vi "Lambda Flow Auto (Read).vi"(6 "ISOBUS address":T5=-1 caption="ISOBUS address (-1)", 8 "error in":errorcluster, 11 "Mercury Reference In":T2) -> (0 "error out":errorcluster, 2 "Lambda Auto":string, 3 "Mercury Reference Out":T2, 4 "Valid?":T1)   [LabVIEW 2016, in "Mercury iXX.lvlib" / "Lambda.lvlib"]
doc: "Check if the flow of the control loop is in automatic mode."
uses:
  Lambda.lvlib
  Controls/Mercury Reference.ctl
  Controls/Comms Transport Layer.ctl
  Private/Controls/Query Dynamic Reference.ctl
  Controls/ISOBus Address.ctl
  Controls/Is Valid LED.ctl
  Private/Controls/Command Verbs.ctl
  Mercury iXX.lvlib
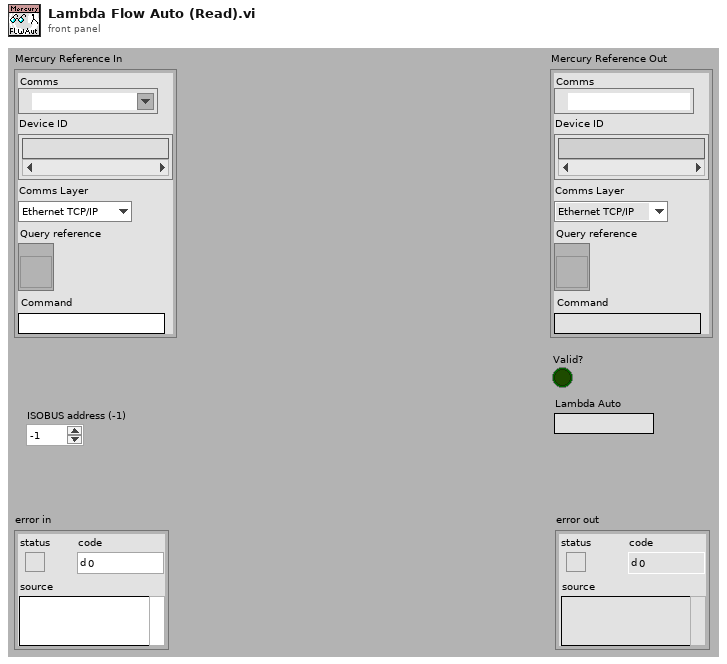
[diagram p1: front panel]
types:
  T1 = typedef "Mercury iXX.lvlib/Is Valid LED.ctl" = bool
  T2 = typedef "Mercury iXX.lvlib/Mercury Reference.ctl" = cluster{"Comms":refnum<visa-resource-name>, "Device ID":string[], "Comms Layer":T3, "Command":string, "Query reference":T4}
  T3 = typedef "Mercury iXX.lvlib/Comms Transport Layer.ctl" = enum16{"Ethernet TCP/IP", "USB", "ISOBus - RS-232", "GPIB"}
  T4 = typedef "Mercury iXX.lvlib/Query Dynamic Reference.ctl" = refnum<vi>
  T5 = typedef "Mercury iXX.lvlib/ISOBus Address.ctl" = i32
  T6 = typedef "Mercury iXX.lvlib/Command Verbs.ctl" = string
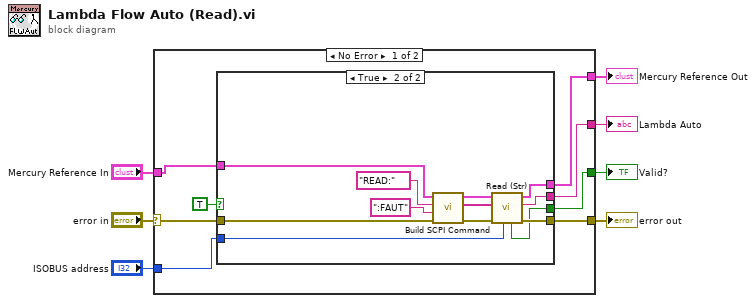
[diagram p0: block diagram]
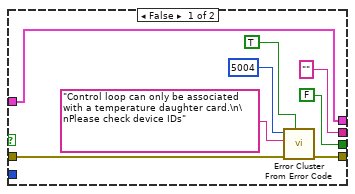
[diagram p2: hidden frame]
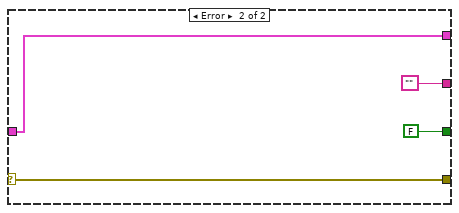
[diagram p3: hidden frame]
diagram:
  n1 = case shown="No Error" "error in" {
    selector: "error in" -> [w8 w38]
    tunnel: "Mercury Reference In" -> [w9 w39]
    tunnel: [w15 w39] -> w1
    tunnel: [w13 w38] -> w2
    tunnel: "ISOBUS address" -> [w14 _]
    tunnel: [w12 T1 FALSE ("Valid?")] -> w4
    tunnel: [w11 ""] -> w3
    frame No Error {
      n2 = case shown="True" TRUE {
        tunnel: w9 -> [w23 w29]
        tunnel: [w23 w24] -> w15
        tunnel: w8 -> [w21 w30]
        tunnel: w14 -> [_ w27]
        tunnel: [w22 w28] -> w13
        tunnel: [T1 FALSE ("Valid?") w26] -> w12
        tunnel: ["" ("Response") w25] -> w11
        frame False {
          n3 = call <vilib>:"Error Cluster From Error Code.vi"("show call chain? (False)"=TRUE, "error in (no error)"=w21, "error message (\"\")"="Control loop can only be associated with a temperature daughter card.\n\nPlease check device IDs" ("error message (\"\")"), "error code (0)"=5004) -> ("error out"=w22:errorcluster)  [unwired: 5 out]
        }
        frame True {
          n4 = call "Build SCPI Command.vi"("error in"=w30, "Noun(s)"=":FAUT" ("Command"), "Verb"=T6 "READ:", "Mercury Reference In"=w29) -> ("error out"=w31:errorcluster, "SCPI Message(s)"=w34:string[], "Mercury Reference Out"=w33:T2)  [unwired: 5 out]
          n5 = call "Read (Str).vi"("ISOBUS address"=w27, "error in"=w31, "SCPI Message(s)"=w34, "Mercury Reference In"=w33) -> ("error out"=w28:errorcluster, "Response"=w25:string, "Mercury Reference Out"=w24:T2, "Valid?"=w26:T1)  [unwired: 4 out]
        }
      }
    }
    frame Error {
    }
  }
  "Mercury Reference Out" <- w1
  "Lambda Auto" <- w3
  "error out" <- w2
  "Valid?" <- w4
